vi "Maxi Gauge-Get Pressure,Status.vi"(8 "Fehler (Eingang, kein Fehler)":errorcluster, 9 "Sensor Nr.:":i32(ring) items=["sensor 1", "sensor 2", "sensor 3", "sensor 4", "sensor 5", "sensor 6"], 10 "Node address":i8=-1 min=-1 max=31 step=1, 11 "VISA-Ressource in":refnum<visa-resource-name>) -> (0 "Fehler (Ausgang)":errorcluster, 1 "Pressure":dbl format="%.3e", 2 "Status":i32(ring) items=["data OK", "underrange", "overrange", "sensor error", "sensor off", "no sensor", "ID error"], 3 "VISA-Ressource out":refnum<visa-resource-name>)   [LabVIEW 2018, in "Maxi Gauge.lvlib"]
uses:
  Maxi Gauge.lvlib
panel:
  # "mbar"
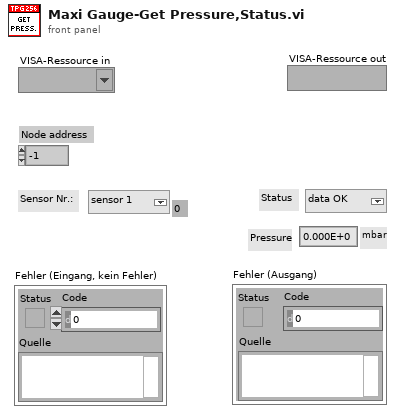
[diagram p1: front panel]
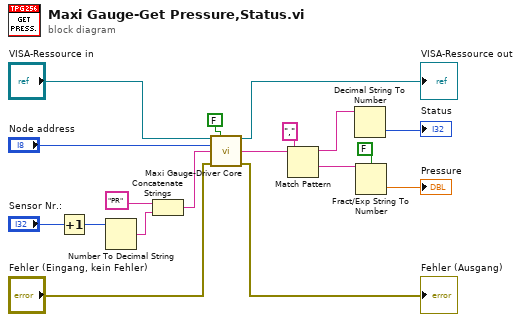
[diagram p0: block diagram]
diagram:
  n1 = Increment(x="Sensor Nr.:") -> (x+1=w17:i32)
  n2 = Number To Decimal String(number=w17) -> (decimal integer string=w12:string)  [unwired: 1 in]
  n3 = Concatenate Strings("PR", w12) -> (w7:string)
  n4 = call "Maxi Gauge-Driver Core.vi"("VISA-Ressource in"="VISA-Ressource in", "Write/Read"=FALSE, "Node address"="Node address", "Command"=w7, "Fehler (Eingang)"="Fehler (Eingang, kein Fehler)") -> ("VISA-Ressource out"=→"VISA-Ressource out":refnum<visa-resource-name>, "String Out"=w1:string, "Fehler (Ausgang)"=→"Fehler (Ausgang)":errorcluster)  [unwired: 8 in]
  n5 = Match Pattern(string=w1, regular expression=",") -> (before substring=w9:string, after substring=w10:string)  [unwired: 1 in, 2 out]
  n6 = Decimal String To Number(string=w9) -> (number=→"Status":i32)  [unwired: 2 in, 1 out]
  n7 = Fract/Exp String To Number(use system decimal point (T)=FALSE ("Systemdezimalzeichen verwenden (T)"), string=w10) -> (number=→"Pressure":dbl)  [unwired: 2 in, 1 out]
